vi "Parse Disk Info.vi"(4 "Result":string="Filesystem     1K-blocks     Used Available Use% Mounted on\n/dev/root        3508400  2415784    893960  73% /\ndevtmpfs         1923988        0   1923988   0% /dev\ntmpfs            1926044      252   1925792   1% /run\ntmpfs            1001544    12704    988840   2% /var/volatile\n/dev/sda2         168903    55539    100749  36% /boot\n/dev/sda3          13129     4415      7639  37% /etc/natinst/share\n/dev/mmcblk0p1  31154688 23226368   7928320  75% /media/mmcblk0p1") -> (7 "Disk Map":map{string, T1}(c390))   [LabVIEW 2020, in "Volatus.lvlib" / "Linux System SAL.lvclass"]
uses:
  Linux System SAL.lvclass
  Disk Info.ctl
  <vilib>/Utility/error.llb/whitespace.ctl
  Linux System SAL.lvclass/Linux System SAL.ctl
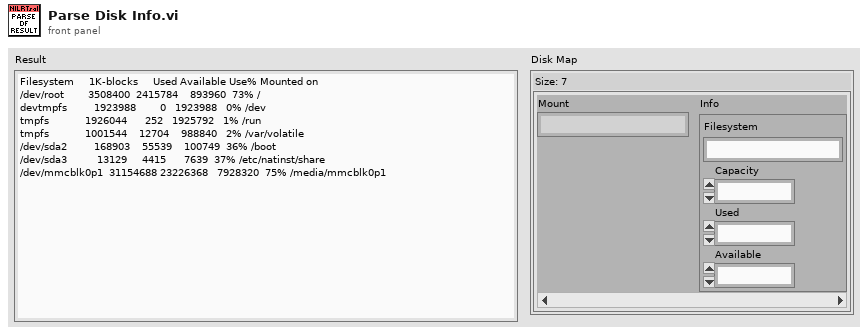
[diagram p1: front panel]
types:
  T1 = typedef "Volatus.lvlib/Linux System SAL.lvclass/Disk Info.ctl" = cluster{"Filesystem":string, "Capacity":dbl, "Used":dbl, "Available":dbl}
  T2 = typedef "whitespace.ctl" = u16
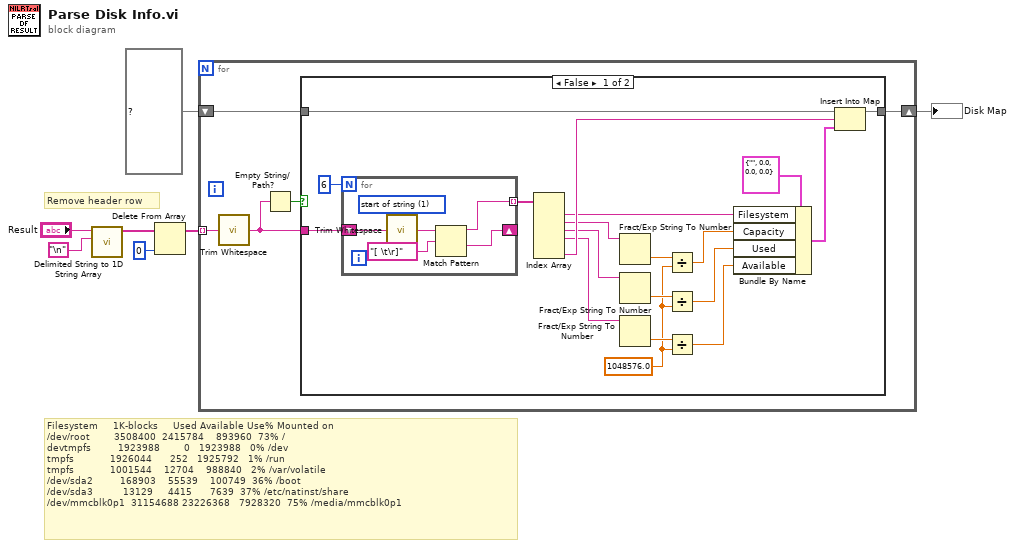
[diagram p0: block diagram]
diagram:
  # "Remove header row"
  # "Filesystem     1K-blocks     Used Available Use% Mounted on\n/dev/root        3508400  2415784    893960  73% /\ndevtmpfs         1923988        0   1923988   0% /dev\ntmpfs            1926044      252   1925792   1% /run\ntmpfs            1001544    12704    988840   2% /var/volatile\n/dev/sda2         168903    55539    100749  36% /boot\n/dev/sda3          13129     4415      7639  37% /etc/natinst/share\n/dev/mmcblk0p1  31154688 23226368   7928320  75% /media/mmcblk0p1"
  n1 = call <vilib>:"Delimited String to 1D String Array.vi"("delimiter"="\n", "delimited string"="Result") -> ("string array"=w5:string[])  [unwired: 9 in]
  n2 = Delete From Array(array=w5, index=0) -> (array with subset deleted=w2:string[])  [unwired: 1 in, 1 out]
  n3 = for {
    tunnel: w2 -> [w10] mode=indexing
    shift-right: [w12] -> w1
    shift-left: map{string, T1} {} ("Disk Map") -> [w11]
    n4 = call <vilib>:"Trim Whitespace.vi"("string"=w10) -> ("trimmed string"=w8:string)  [unwired: 1 in]
    n5 = Empty String/Path?(string/path=w8) -> (empty?=w9:bool)
    n6 = case shown="False" w9 {
      tunnel: [w29 w38] -> w12
      tunnel: w11 -> [w28 w38]
      tunnel: w8 -> [w23 _]
      frame False {
        w20 = 1048576.0
        n7 = for {
          N: 6 -> [_]
          shift-right: [w32] -> _
          shift-left: w23 -> [w37]
          tunnel: [w33] -> w30 mode=indexing
          w36 = T2 1 items=["both", "start of string", "end of string"] ("location (both)")
          n8 = call <vilib>:"Trim Whitespace.vi"("string"=w37, "location (both)"=w36) -> ("trimmed string"=w35:string)
          n9 = Match Pattern(string=w35, regular expression="[ \t\r]") -> (before substring=w33:string, after substring=w32:string)  [unwired: 1 in, 2 out]
        }
        n10 = Index Array(array=w30) -> (element #1=w19:string, element #2=w18:string, element #3=w16:string, element #4=w14:string, element #6=w22:string)  [unwired: 6 in, 1 out]
        n11 = Fract/Exp String To Number(string=w18) -> (number=w26:dbl)  [unwired: 3 in, 1 out]
        n12 = Fract/Exp String To Number(string=w16) -> (number=w25:dbl)  [unwired: 3 in, 1 out]
        n13 = Fract/Exp String To Number(string=w14) -> (number=w21:dbl)  [unwired: 3 in, 1 out]
        n14 = Divide(x=w26, y=w20) -> (x/y=w17:dbl)
        n15 = Divide(x=w25, y=w20) -> (x/y=w15:dbl)
        n16 = Divide(x=w21, y=w20) -> (x/y=w13:dbl)
        n17 = Bundle By Name(cluster=T1 {"Filesystem"="", "Capacity"=0.0, "Used"=0.0, "Available"=0.0} ("Disk Info"), "Filesystem"=w19, "Capacity"=w17, "Used"=w15, "Available"=w13) -> (w24:T1)
        n18 = Insert Into Map(map in=w28, key=w22, value=w24) -> (map out=w29:map{string, T1})  [unwired: 2 out]
      }
      frame True {
      }
    }
  }
  "Disk Map" <- w1
